vi "Log events FGV.vi"(6 "action":T2, 8 "error in (no error)":errorcluster, 10 "Event data":variant, 11 "Log event":T1) -> (0 "error out":errorcluster)   [LabVIEW 2014]
doc: "Log file functional global variable\nwith following actions:\n\n<B>-open log file:</B> Opens CSV log file in main Boiler aplication folder\n<B>-log event:</B> Logs event time , event name and parameters to CSV file\n<B>-close file :</B> Closes CSV log file"
uses:
  Controls/Log file FGV action enum.ctl
  Controls/Log event enum.ctl
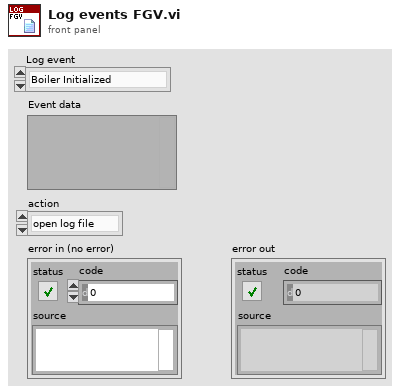
[diagram p1: front panel]
types:
  T1 = typedef "Log event enum.ctl" = enum16{"Boiler Initialized", "Boiler Ready", "Start Pre-Purge", "Pre-Purge Complete", "Pilot ON", "Pilot proved", "Forced Draft Fan ON", "Boiler Running", "Start Shutdown Purge", "Shutdown Purge Complete"}
  T2 = typedef "Log file FGV action enum.ctl" = enum16{"open log file", "log event", "close log file"}
  T3 = enum16{"open", "replace", "create", "open or create", "replace or create", "replace or create with confirmation"}
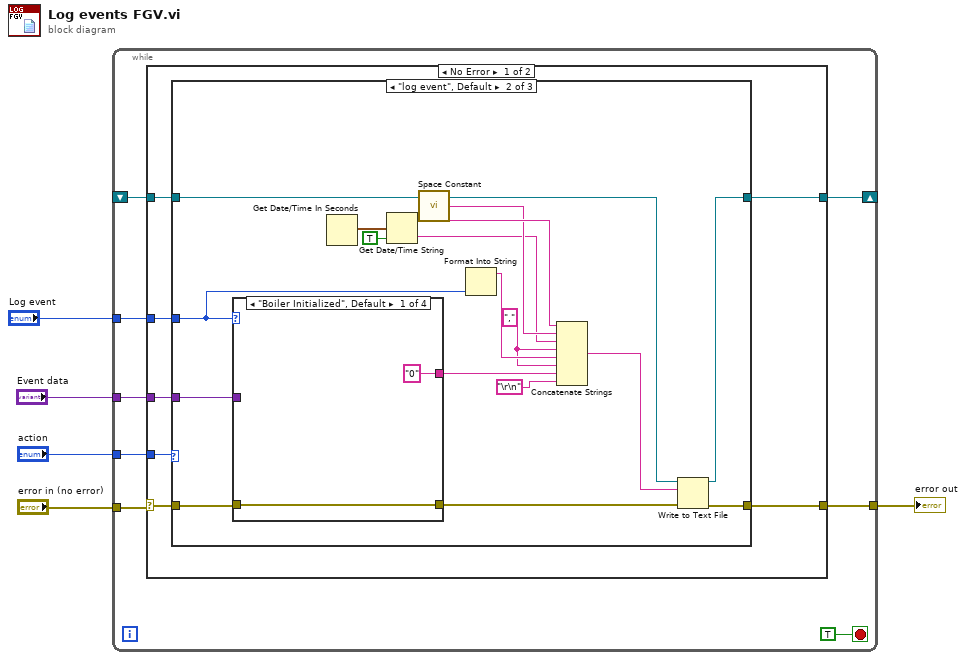
[diagram p0: block diagram]
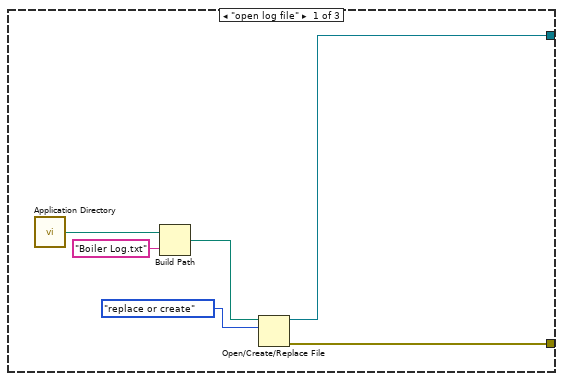
[diagram p2: hidden frame]
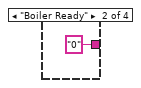
[diagram p3: hidden frame]
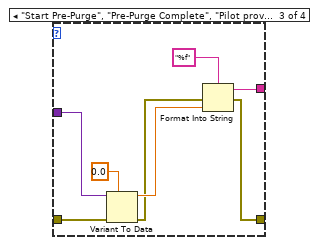
[diagram p4: hidden frame]
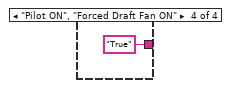
[diagram p5: hidden frame]
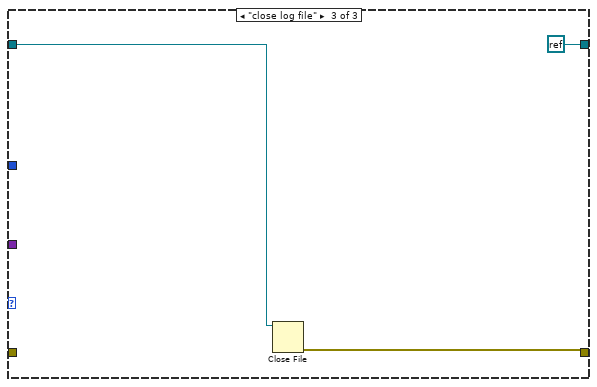
[diagram p6: hidden frame]
diagram:
  n1 = while {
    tunnel: "action" -> [w12]
    tunnel: "error in (no error)" -> [w11]
    tunnel: [w10] -> w3
    shift-right: [w9] -> _
    shift-left: _ -> [w8]
    tunnel: "Log event" -> [w7]
    tunnel: "Event data" -> [w6]
    stop <- TRUE stop-if-true
    n2 = case shown="No Error" w11 {
      selector: w11 -> [w14 w60]
      tunnel: w12 -> [w20 _]
      tunnel: [w19 w60] -> w10
      tunnel: [w18 w59] -> w9
      tunnel: w8 -> [w17 w59]
      tunnel: w7 -> [w16 _]
      tunnel: w6 -> [w15 _]
      frame No Error {
        n3 = case shown="\"log event\", Default" w20 {
          tunnel: [w22 w27 w56] -> w19
          tunnel: [w21 w28 refnum<k0> refnum] -> w18
          tunnel: w17 -> [_ w29 w57]
          tunnel: w16 -> [_ w38 _]
          tunnel: w15 -> [_ w35 _]
          tunnel: w14 -> [_ w34 _]
          frame "open log file" {
            n4 = call <vilib>:"Application Directory.vi"() -> ("Application Directory"=w26:path)
            n5 = Build Path(base path=w26, name or relative path="Boiler Log.txt") -> (appended path=w24:path)
            n6 = Open/Create/Replace File(file path (use dialog)=w24, operation (0:open)=T3."replace or create") -> (refnum out=w21:refnum<file>, error out=w22:errorcluster)  [unwired: 4 in, 1 out]
          }
          frame "log event", Default {
            w36 = ","
            n7 = case shown="\"Boiler Initialized\", Default" w38 {
              tunnel: w35 -> [_ _ w53 _]
              tunnel: w34 -> [w44 _ w54 _]
              tunnel: ["0" "0" w51 "True"] -> w33
              tunnel: [w44 _ w48 _] -> w31
              frame "Boiler Initialized", Default {
              }
              frame "Boiler Ready" {
              }
              frame "Start Pre-Purge", "Pre-Purge Complete", "Pilot proved", "Boiler Running".."Shutdown Purge Complete" {
                n8 = Variant To Data(error in=w54, type=0.0, Variant=w53) -> (data=w50:dbl, error out=w49:errorcluster)
                n9 = Format Into String(format string="%f", error in=w49, w50) -> (resulting string=w51:string, error out=w48:errorcluster)  [unwired: 1 in]
              }
              frame "Pilot ON", "Forced Draft Fan ON" {
              }
            }
            n10 = Get Date/Time In Seconds() -> (seconds since 1Jan1904=w43:timestamp)
            n11 = Get Date/Time String(seconds (now)=w43, want seconds? (F)=TRUE) -> (date string=w41:string, time string=w39:string)  [unwired: 1 in]
            n12 = call <vilib>:"Space Constant.vi"() -> ("String"=w40:string)
            n13 = Format Into String(w38) -> (resulting string=w37:string)  [unwired: 3 in, 1 out]
            n14 = Concatenate Strings(w41, w40, w39, w36, w37, w36, w33, "\r\n") -> (w30:string)
            n15 = Write to Text File(file (use dialog)=w29, text=w30, error in=w31) -> (refnum out=w28:refnum<file>, error out=w27:errorcluster)  [unwired: 1 in, 1 out]
          }
          frame "close log file" {
            n16 = Close File(refnum=w57) -> (error out=w56:errorcluster)  [unwired: 1 in, 1 out]
          }
        }
      }
      frame Error {
      }
    }
  }
  "error out" <- w3
